vi "Count True Elements.vi"(4 "Array":bool[](array[boolean])) -> (1 "Numeric":u32)   [LabVIEW 2013, in "Empirical Mode Decomposition.lvlib"]
uses:
  Empirical Mode Decomposition.lvlib
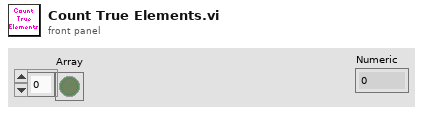
[diagram p1: front panel]
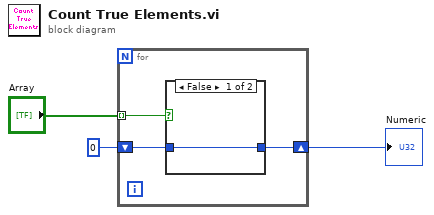
[diagram p0: block diagram]
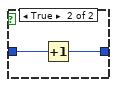
[diagram p2: hidden frame]
diagram:
  n1 = for {
    tunnel: "Array" -> [w6] mode=indexing
    shift-right: [w4] -> w1
    shift-left: 0 -> [w5]
    n2 = case shown="False" w6 {
      tunnel: w5 -> [w7 w9]
      tunnel: [w7 w8] -> w4
      frame False {
      }
      frame True {
        n3 = Increment(x=w9) -> (x+1=w8:i32)
      }
    }
  }
  "Numeric" <- w1
